vi "export_DFD.vi"(11 "dfd file name":string) -> ()   [LabVIEW 2013]
uses:
  FT_HMI.llb/GLOBAL_GEN.vi
  FT_HMI.llb/GLOBAL_PUMPS_PARAMS.vi
panel:
  in  "index":i32
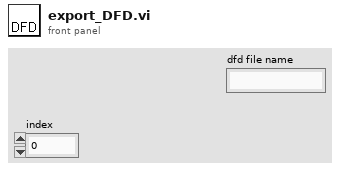
[diagram p1: front panel]
types:
  T1 = cluster{"VAC":cluster{"ENABLE":bool, "PUMPING_TIME [ms]":dbl, "MEASUREMENT_TIME [ms]":dbl, "PRESSURE_LIMIT [bar]":sgl}, "Q1":cluster{"ENABLE":bool, "PUMPING_TIME  [ms]":dbl, "MEASUREMENT_TIME  [ms]":sgl, "FLOW_TARGET  [ml/min]":sgl, "FLOW_LIMIT_UP  [ml/min]":sgl, "FLOW_LIMIT_DOWN [ml/min]":sgl, "PRESSURE_TARGET [bar]":sgl, "PRESSURE_LIMIT_UP [bar]":sgl, "PRESSURE_LIMIT_DOWN [bar]":sgl, "MAX_FLOW":bool}, "Q2":cluster{"ENABLE":bool, "PUMPING_TIME [ms]":dbl, "MEASUREMENT_TIME [ms]":dbl, "FLOW_TARGET [ml/min]":sgl, "FLOW_LIMIT_UP [ml/min]":sgl, "FLOW_LIMIT_DOWN [ml/min]":sgl, "PRESSURE_TARGET [bar]":sgl, "PRESSURE_LIMIT_UP [bar]":sgl, "PRESSURE_LIMIT_DOWN [bar]":sgl, "MAX_FLOW":bool}, "PMAX":cluster{"ENABLE":bool, "PUMPING_TIME [ms]":dbl, "MEASUREMENT_TIME [ms]":dbl, "PRESSURE_LIMIT [bar]":sgl, "PRESSURE_LOOSE_TIME [ms]":sgl, "PRESSURE_LOOSE [mbar]":sgl}, "PRINT":cluster{"ENABLE":bool}, "SUPPLY":cluster{"VOLTAGE [V]":dbl, "FREQUENCY [Hz]":dbl}}
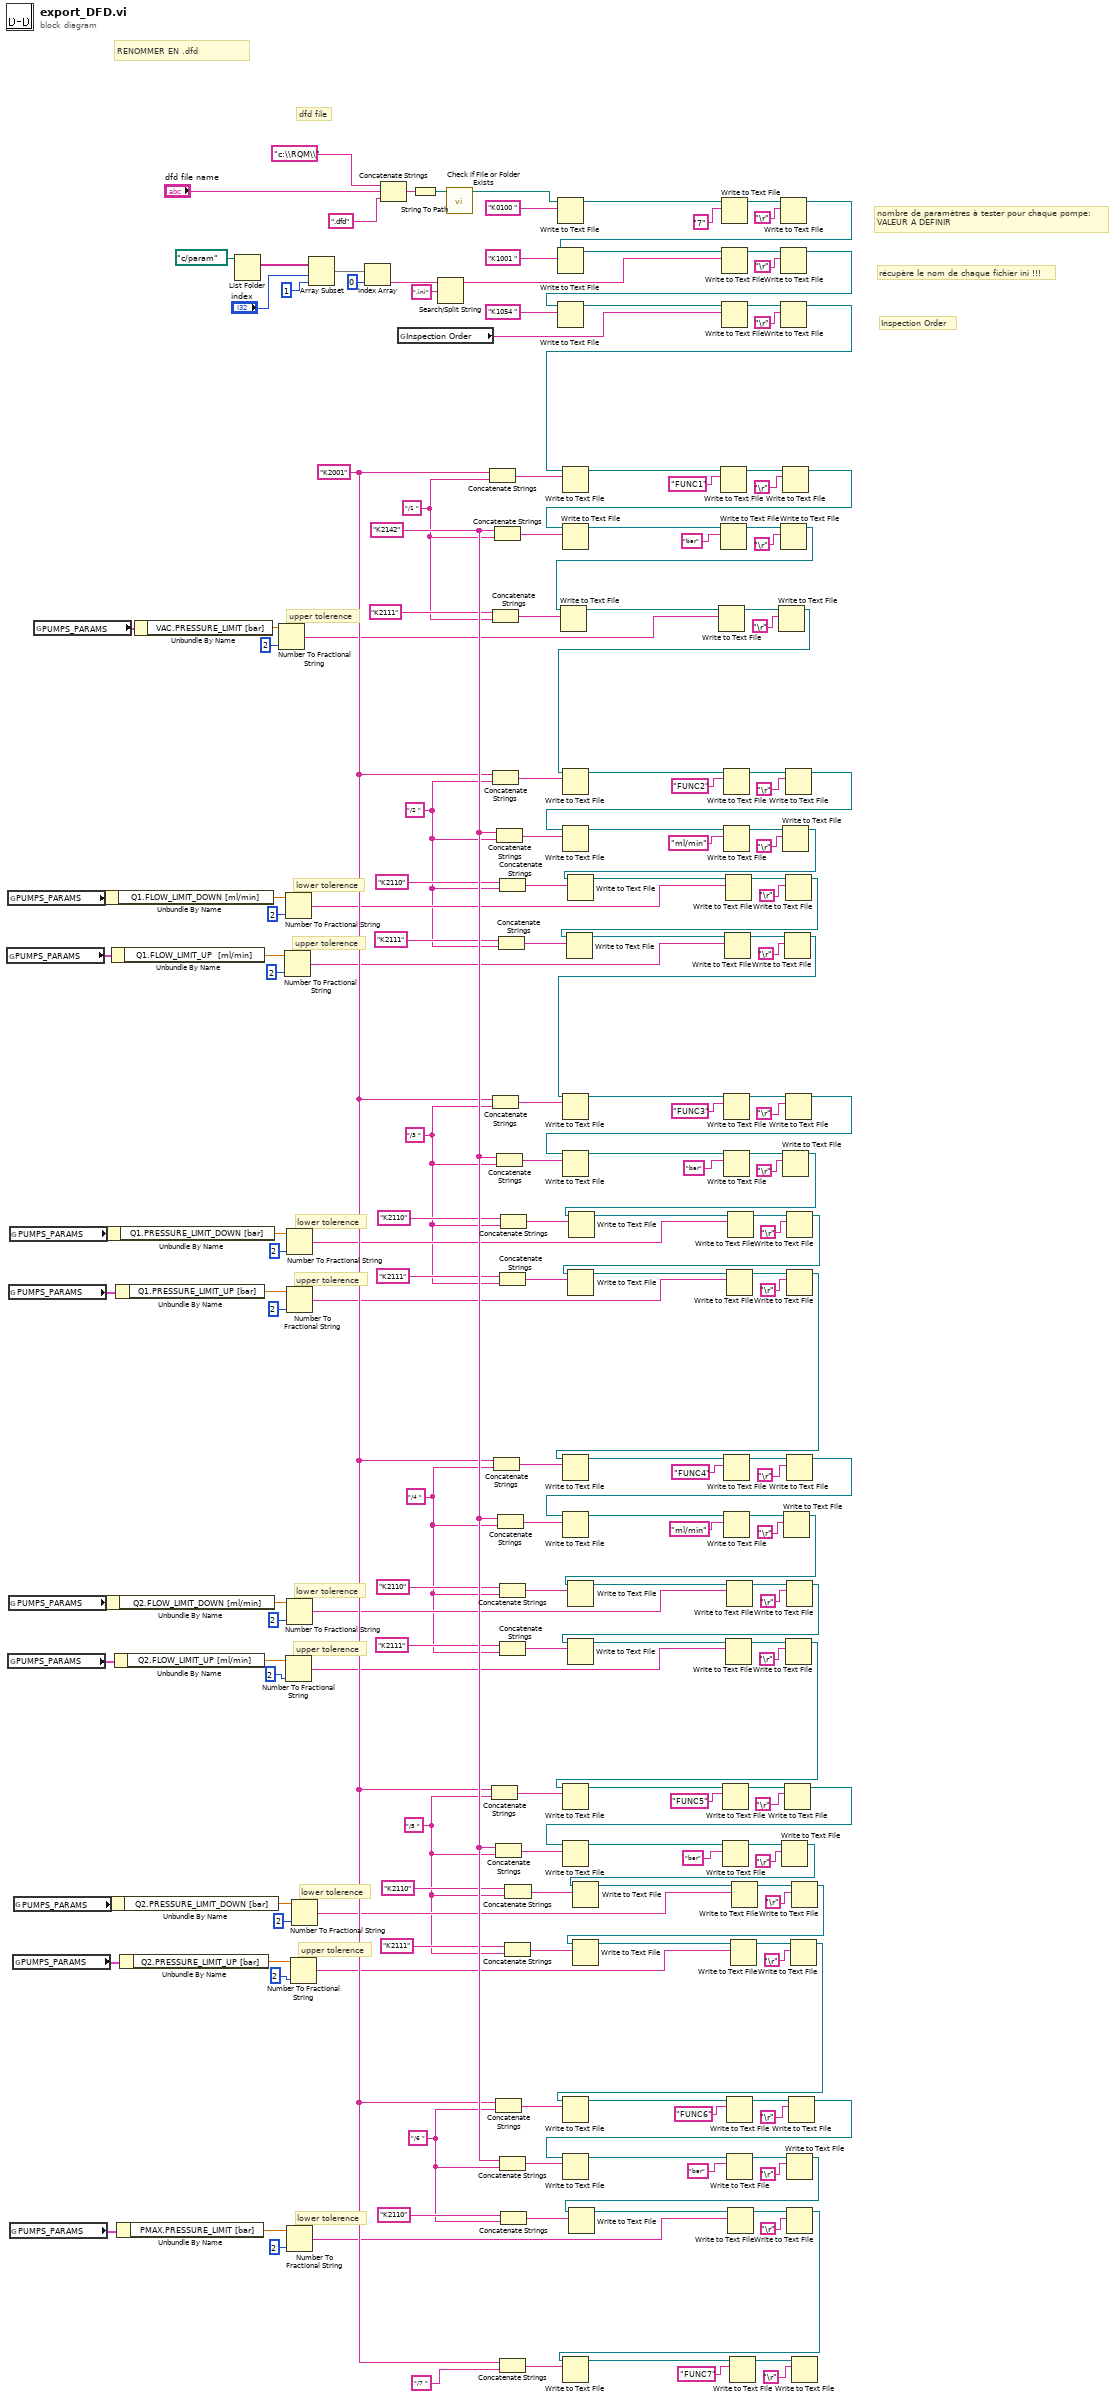
[diagram p0: block diagram]
diagram:
  w2 = "/6 " ("string")
  w1 = "/5 " ("string")
  w43 = "/4 " ("string")
  w63 = "/3 " ("string")
  w84 = "/2 " ("string")
  w114 = "K2142" ("text")
  w108 = "/1 " ("string")
  w104 = "K2001" ("text")
  # "lower tolerence"
  # "upper tolerence"
  # "lower tolerence"
  # "upper tolerence"
  # "lower tolerence"
  # "upper tolerence"
  # "lower tolerence"
  # "upper tolerence"
  # "lower tolerence"
  # "upper tolerence"
  # "RENOMMER EN .dfd"
  # "récupère le nom de chaque fichier ini !!!"
  # "Inspection Order"
  # "dfd file"
  # "nombre de paramètres à tester pour chaque pompe:\nVALEUR A DEFINIR"
  n1 = global read "GLOBAL_PUMPS_PARAMS.vi" "PUMPS_PARAMS"() -> (w87:T1)
  n2 = global read "GLOBAL_PUMPS_PARAMS.vi" "PUMPS_PARAMS"() -> (w98:T1)
  n3 = global read "GLOBAL_PUMPS_PARAMS.vi" "PUMPS_PARAMS"() -> (w47:T1)
  n4 = global read "GLOBAL_PUMPS_PARAMS.vi" "PUMPS_PARAMS"() -> (w77:T1)
  n5 = global read "GLOBAL_PUMPS_PARAMS.vi" "PUMPS_PARAMS"() -> (w58:T1)
  n6 = global read "GLOBAL_PUMPS_PARAMS.vi" "PUMPS_PARAMS"() -> (w66:T1)
  n7 = global read "GLOBAL_PUMPS_PARAMS.vi" "PUMPS_PARAMS"() -> (w11:T1)
  n8 = global read "GLOBAL_PUMPS_PARAMS.vi" "PUMPS_PARAMS"() -> (w29:T1)
  n9 = global read "GLOBAL_PUMPS_PARAMS.vi" "PUMPS_PARAMS"() -> (w18:T1)
  n10 = global read "GLOBAL_PUMPS_PARAMS.vi" "PUMPS_PARAMS"() -> (w106:T1)
  n11 = Unbundle By Name(w98) -> ("Q1.FLOW_LIMIT_DOWN [ml/min]"=w99:sgl)
  n12 = Unbundle By Name(w58) -> ("Q2.FLOW_LIMIT_DOWN [ml/min]"=w59:sgl)
  n13 = Unbundle By Name(w66) -> ("Q1.PRESSURE_LIMIT_DOWN [bar]"=w65:sgl)
  n14 = Unbundle By Name(w87) -> ("Q1.FLOW_LIMIT_UP  [ml/min]"=w86:sgl)
  n15 = Unbundle By Name(w18) -> ("Q2.PRESSURE_LIMIT_DOWN [bar]"=w17:sgl)
  n16 = Unbundle By Name(w47) -> ("Q2.FLOW_LIMIT_UP [ml/min]"=w46:sgl)
  n17 = Unbundle By Name(w77) -> ("Q1.PRESSURE_LIMIT_UP [bar]"=w78:sgl)
  n18 = Unbundle By Name(w11) -> ("PMAX.PRESSURE_LIMIT [bar]"=w12:sgl)
  n19 = Unbundle By Name(w29) -> ("Q2.PRESSURE_LIMIT_UP [bar]"=w30:sgl)
  n20 = Unbundle By Name(w106) -> ("VAC.PRESSURE_LIMIT [bar]"=w103:sgl)
  n21 = List Folder(path=path "c:/param") -> (filenames=w185:string[])  [unwired: 3 in, 3 out]
  n22 = Number To Fractional String(number=w103, precision (6)=i16 2) -> (F-format string=w102:string)  [unwired: 2 in]
  n23 = Number To Fractional String(number=w86, precision (6)=i16 2) -> (F-format string=w85:string)  [unwired: 2 in]
  n24 = Number To Fractional String(number=w99, precision (6)=i16 2) -> (F-format string=w100:string)  [unwired: 2 in]
  n25 = Number To Fractional String(number=w46, precision (6)=i16 2) -> (F-format string=w45:string)  [unwired: 2 in]
  n26 = Number To Fractional String(number=w78, precision (6)=i16 2) -> (F-format string=w79:string)  [unwired: 2 in]
  n27 = Number To Fractional String(number=w59, precision (6)=i16 2) -> (F-format string=w60:string)  [unwired: 2 in]
  n28 = Number To Fractional String(number=w65, precision (6)=i16 2) -> (F-format string=w64:string)  [unwired: 2 in]
  n29 = Number To Fractional String(number=w12, precision (6)=i16 2) -> (F-format string=w13:string)  [unwired: 2 in]
  n30 = Number To Fractional String(number=w30, precision (6)=i16 2) -> (F-format string=w31:string)  [unwired: 2 in]
  n31 = Number To Fractional String(number=w17, precision (6)=i16 2) -> (F-format string=w16:string)  [unwired: 2 in]
  n32 = Array Subset(array=w185, index="index", length=1) -> (w183:string[])
  n33 = Index Array(array=w183, index=0) -> (element=w179:string)
  n34 = Concatenate Strings("c:\\RQM\\", "dfd file name", ".dfd") -> (w215:string)
  n35 = global read "GLOBAL_GEN.vi" "Inspection Order"() -> (w188:string)
  n36 = String To Path(string=w215) -> (path=w217:path)
  n37 = Search/Split String(string=w179, search string/char (-)=".ini") -> (substring before match=w178:string)  [unwired: 1 in, 2 out]
  n38 = call <vilib>:"Check if File or Folder Exists.vi"("path"=w217) -> ("dup path"=w213:path)  [unwired: 8 in, 2 out]
  n39 = Concatenate Strings(w104, w108) -> (w190:string)
  n40 = Concatenate Strings(w104, w1) -> (w134:string)
  n41 = Concatenate Strings("K2111" ("text"), w108) -> (w112:string)
  n42 = Concatenate Strings(w104, w84) -> (w167:string)
  n43 = Concatenate Strings(w104, w63) -> (w156:string)
  n44 = Concatenate Strings(w104, w43) -> (w145:string)
  n45 = Concatenate Strings(w114, w108) -> (w189:string)
  n46 = Concatenate Strings(w114, w1) -> (w133:string)
  n47 = Concatenate Strings(w104, w2) -> (w123:string)
  n48 = Concatenate Strings(w114, w84) -> (w166:string)
  n49 = Concatenate Strings(w114, w63) -> (w155:string)
  n50 = Concatenate Strings(w114, w43) -> (w144:string)
  n51 = Concatenate Strings("K2111" ("text"), w84) -> (w91:string)
  n52 = Concatenate Strings("K2110" ("text"), w84) -> (w94:string)
  n53 = Concatenate Strings("K2111" ("text"), w43) -> (w51:string)
  n54 = Concatenate Strings(w104, "/7 " ("string")) -> (w116:string)
  n55 = Concatenate Strings("K2111" ("text"), w63) -> (w73:string)
  n56 = Concatenate Strings("K2110" ("text"), w43) -> (w54:string)
  n57 = Concatenate Strings(w114, w2) -> (w122:string)
  n58 = Concatenate Strings("K2110" ("text"), w63) -> (w70:string)
  n59 = Concatenate Strings("K2110" ("text"), w2) -> (w7:string)
  n60 = Concatenate Strings("K2111" ("text"), w1) -> (w25:string)
  n61 = Concatenate Strings("K2110" ("text"), w1) -> (w22:string)
  n62 = Write to Text File(file (use dialog)=w213, text="K0100 ") -> (refnum out=w211:refnum<file>)  [unwired: 2 in, 2 out]
  n63 = Write to Text File(file (use dialog)=w211, text="7") -> (refnum out=w210:refnum<file>)  [unwired: 2 in, 2 out]
  n64 = Write to Text File(file (use dialog)=w210, text="\r") -> (refnum out=w204:refnum<file>)  [unwired: 2 in, 2 out]
  n65 = Write to Text File(file (use dialog)=w204, text="K1001 ") -> (refnum out=w207:refnum<file>)  [unwired: 2 in, 2 out]
  n66 = Write to Text File(file (use dialog)=w207, text=w178) -> (refnum out=w206:refnum<file>)  [unwired: 2 in, 2 out]
  n67 = Write to Text File(file (use dialog)=w206, text="\r") -> (refnum out=w199:refnum<file>)  [unwired: 2 in, 2 out]
  n68 = Write to Text File(file (use dialog)=w199, text="K1054 ") -> (refnum out=w202:refnum<file>)  [unwired: 2 in, 2 out]
  n69 = Write to Text File(file (use dialog)=w202, text=w188) -> (refnum out=w201:refnum<file>)  [unwired: 2 in, 2 out]
  n70 = Write to Text File(file (use dialog)=w201, text="\r") -> (refnum out=w177:refnum<file>)  [unwired: 2 in, 2 out]
  n71 = Write to Text File(file (use dialog)=w177, text=w190) -> (refnum out=w198:refnum<file>)  [unwired: 2 in, 2 out]
  n72 = Write to Text File(file (use dialog)=w198, text="FUNC1") -> (refnum out=w197:refnum<file>)  [unwired: 2 in, 2 out]
  n73 = Write to Text File(file (use dialog)=w197, text="\r") -> (refnum out=w176:refnum<file>)  [unwired: 2 in, 2 out]
  n74 = Write to Text File(file (use dialog)=w176, text=w189) -> (refnum out=w194:refnum<file>)  [unwired: 2 in, 2 out]
  n75 = Write to Text File(file (use dialog)=w194, text="bar") -> (refnum out=w193:refnum<file>)  [unwired: 2 in, 2 out]
  n76 = Write to Text File(file (use dialog)=w193, text="\r") -> (refnum out=w105:refnum<file>)  [unwired: 2 in, 2 out]
  n77 = Write to Text File(file (use dialog)=w105, text=w112) -> (refnum out=w109:refnum<file>)  [unwired: 2 in, 2 out]
  n78 = Write to Text File(file (use dialog)=w109, text=w102) -> (refnum out=w110:refnum<file>)  [unwired: 2 in, 2 out]
  n79 = Write to Text File(file (use dialog)=w110, text="\r") -> (refnum out=w107:refnum<file>)  [unwired: 2 in, 2 out]
  n80 = Write to Text File(file (use dialog)=w107, text=w167) -> (refnum out=w175:refnum<file>)  [unwired: 2 in, 2 out]
  n81 = Write to Text File(file (use dialog)=w175, text="FUNC2") -> (refnum out=w174:refnum<file>)  [unwired: 2 in, 2 out]
  n82 = Write to Text File(file (use dialog)=w174, text="\r") -> (refnum out=w165:refnum<file>)  [unwired: 2 in, 2 out]
  n83 = Write to Text File(file (use dialog)=w165, text=w166) -> (refnum out=w171:refnum<file>)  [unwired: 2 in, 2 out]
  n84 = Write to Text File(file (use dialog)=w171, text="ml/min") -> (refnum out=w170:refnum<file>)  [unwired: 2 in, 2 out]
  n85 = Write to Text File(file (use dialog)=w170, text="\r") -> (refnum out=w83:refnum<file>)  [unwired: 2 in, 2 out]
  n86 = Write to Text File(file (use dialog)=w83, text=w94) -> (refnum out=w97:refnum<file>)  [unwired: 2 in, 2 out]
  n87 = Write to Text File(file (use dialog)=w97, text=w100) -> (refnum out=w96:refnum<file>)  [unwired: 2 in, 2 out]
  n88 = Write to Text File(file (use dialog)=w96, text="\r") -> (refnum out=w82:refnum<file>)  [unwired: 2 in, 2 out]
  n89 = Write to Text File(file (use dialog)=w82, text=w91) -> (refnum out=w88:refnum<file>)  [unwired: 2 in, 2 out]
  n90 = Write to Text File(file (use dialog)=w88, text=w85) -> (refnum out=w89:refnum<file>)  [unwired: 2 in, 2 out]
  n91 = Write to Text File(file (use dialog)=w89, text="\r") -> (refnum out=w81:refnum<file>)  [unwired: 2 in, 2 out]
  n92 = Write to Text File(file (use dialog)=w81, text=w156) -> (refnum out=w164:refnum<file>)  [unwired: 2 in, 2 out]
  n93 = Write to Text File(file (use dialog)=w164, text="FUNC3") -> (refnum out=w163:refnum<file>)  [unwired: 2 in, 2 out]
  n94 = Write to Text File(file (use dialog)=w163, text="\r") -> (refnum out=w154:refnum<file>)  [unwired: 2 in, 2 out]
  n95 = Write to Text File(file (use dialog)=w154, text=w155) -> (refnum out=w160:refnum<file>)  [unwired: 2 in, 2 out]
  n96 = Write to Text File(file (use dialog)=w160, text="bar") -> (refnum out=w159:refnum<file>)  [unwired: 2 in, 2 out]
  n97 = Write to Text File(file (use dialog)=w159, text="\r") -> (refnum out=w62:refnum<file>)  [unwired: 2 in, 2 out]
  n98 = Write to Text File(file (use dialog)=w62, text=w70) -> (refnum out=w67:refnum<file>)  [unwired: 2 in, 2 out]
  n99 = Write to Text File(file (use dialog)=w67, text=w64) -> (refnum out=w68:refnum<file>)  [unwired: 2 in, 2 out]
  n100 = Write to Text File(file (use dialog)=w68, text="\r") -> (refnum out=w80:refnum<file>)  [unwired: 2 in, 2 out]
  n101 = Write to Text File(file (use dialog)=w80, text=w73) -> (refnum out=w76:refnum<file>)  [unwired: 2 in, 2 out]
  n102 = Write to Text File(file (use dialog)=w76, text=w79) -> (refnum out=w75:refnum<file>)  [unwired: 2 in, 2 out]
  n103 = Write to Text File(file (use dialog)=w75, text="\r") -> (refnum out=w61:refnum<file>)  [unwired: 2 in, 2 out]
  n104 = Write to Text File(file (use dialog)=w61, text=w145) -> (refnum out=w153:refnum<file>)  [unwired: 2 in, 2 out]
  n105 = Write to Text File(file (use dialog)=w153, text="FUNC4") -> (refnum out=w152:refnum<file>)  [unwired: 2 in, 2 out]
  n106 = Write to Text File(file (use dialog)=w152, text="\r") -> (refnum out=w143:refnum<file>)  [unwired: 2 in, 2 out]
  n107 = Write to Text File(file (use dialog)=w143, text=w144) -> (refnum out=w149:refnum<file>)  [unwired: 2 in, 2 out]
  n108 = Write to Text File(file (use dialog)=w149, text="ml/min") -> (refnum out=w148:refnum<file>)  [unwired: 2 in, 2 out]
  n109 = Write to Text File(file (use dialog)=w148, text="\r") -> (refnum out=w42:refnum<file>)  [unwired: 2 in, 2 out]
  n110 = Write to Text File(file (use dialog)=w42, text=w54) -> (refnum out=w57:refnum<file>)  [unwired: 2 in, 2 out]
  n111 = Write to Text File(file (use dialog)=w57, text=w60) -> (refnum out=w56:refnum<file>)  [unwired: 2 in, 2 out]
  n112 = Write to Text File(file (use dialog)=w56, text="\r") -> (refnum out=w44:refnum<file>)  [unwired: 2 in, 2 out]
  n113 = Write to Text File(file (use dialog)=w44, text=w51) -> (refnum out=w48:refnum<file>)  [unwired: 2 in, 2 out]
  n114 = Write to Text File(file (use dialog)=w48, text=w45) -> (refnum out=w49:refnum<file>)  [unwired: 2 in, 2 out]
  n115 = Write to Text File(file (use dialog)=w49, text="\r") -> (refnum out=w41:refnum<file>)  [unwired: 2 in, 2 out]
  n116 = Write to Text File(file (use dialog)=w41, text=w134) -> (refnum out=w142:refnum<file>)  [unwired: 2 in, 2 out]
  n117 = Write to Text File(file (use dialog)=w142, text="FUNC5") -> (refnum out=w141:refnum<file>)  [unwired: 2 in, 2 out]
  n118 = Write to Text File(file (use dialog)=w141, text="\r") -> (refnum out=w132:refnum<file>)  [unwired: 2 in, 2 out]
  n119 = Write to Text File(file (use dialog)=w132, text=w133) -> (refnum out=w138:refnum<file>)  [unwired: 2 in, 2 out]
  n120 = Write to Text File(file (use dialog)=w138, text="bar") -> (refnum out=w137:refnum<file>)  [unwired: 2 in, 2 out]
  n121 = Write to Text File(file (use dialog)=w137, text="\r") -> (refnum out=w15:refnum<file>)  [unwired: 2 in, 2 out]
  n122 = Write to Text File(file (use dialog)=w15, text=w22) -> (refnum out=w19:refnum<file>)  [unwired: 2 in, 2 out]
  n123 = Write to Text File(file (use dialog)=w19, text=w16) -> (refnum out=w20:refnum<file>)  [unwired: 2 in, 2 out]
  n124 = Write to Text File(file (use dialog)=w20, text="\r") -> (refnum out=w32:refnum<file>)  [unwired: 2 in, 2 out]
  n125 = Write to Text File(file (use dialog)=w32, text=w25) -> (refnum out=w28:refnum<file>)  [unwired: 2 in, 2 out]
  n126 = Write to Text File(file (use dialog)=w28, text=w31) -> (refnum out=w27:refnum<file>)  [unwired: 2 in, 2 out]
  n127 = Write to Text File(file (use dialog)=w27, text="\r") -> (refnum out=w14:refnum<file>)  [unwired: 2 in, 2 out]
  n128 = Write to Text File(file (use dialog)=w14, text=w123) -> (refnum out=w131:refnum<file>)  [unwired: 2 in, 2 out]
  n129 = Write to Text File(file (use dialog)=w131, text="FUNC6") -> (refnum out=w130:refnum<file>)  [unwired: 2 in, 2 out]
  n130 = Write to Text File(file (use dialog)=w130, text="\r") -> (refnum out=w121:refnum<file>)  [unwired: 2 in, 2 out]
  n131 = Write to Text File(file (use dialog)=w121, text=w122) -> (refnum out=w127:refnum<file>)  [unwired: 2 in, 2 out]
  n132 = Write to Text File(file (use dialog)=w127, text="bar") -> (refnum out=w126:refnum<file>)  [unwired: 2 in, 2 out]
  n133 = Write to Text File(file (use dialog)=w126, text="\r") -> (refnum out=w4:refnum<file>)  [unwired: 2 in, 2 out]
  n134 = Write to Text File(file (use dialog)=w4, text=w7) -> (refnum out=w10:refnum<file>)  [unwired: 2 in, 2 out]
  n135 = Write to Text File(file (use dialog)=w10, text=w13) -> (refnum out=w9:refnum<file>)  [unwired: 2 in, 2 out]
  n136 = Write to Text File(file (use dialog)=w9, text="\r") -> (refnum out=w3:refnum<file>)  [unwired: 2 in, 2 out]
  n137 = Write to Text File(file (use dialog)=w3, text=w116) -> (refnum out=w120:refnum<file>)  [unwired: 2 in, 2 out]
  n138 = Write to Text File(file (use dialog)=w120, text="FUNC7") -> (refnum out=w119:refnum<file>)  [unwired: 2 in, 2 out]
  n139 = Write to Text File(file (use dialog)=w119, text="\r") -> ()  [unwired: 2 in, 3 out]
